vi "DAQmxTaskContainerConnect-Com-Exec.vi"(8 "error in (no error)":errorcluster, 9 "data":variant, 10 "ControlQueue":refnum<queue>, 11 "DAQmxTaksContainer_General in":refnum<class "DAQmxTaksContainer_General.lvclass">) -> (0 "error out":errorcluster, 3 "DAQmxTaksContainer_General out":refnum<class "DAQmxTaksContainer_General.lvclass">)   [LabVIEW 2018, in "DAQmxTaksContainer_General.lvclass"]
uses:
  DAQmxTaksContainer_General.lvclass
  dependecies/ControlsVIs/Clusters-def/DAQmx-Reply-Connect-client.ctl
  dependecies/ControlsVIs/Clusters-def/DAQmx-Reply-to-Connect.ctl
  dependecies/ControlsVIs/Clusters-def/SERVER-Commands.ctl
  DAQmxTask.lvclass
  Control/Control-Server/Control-Server.lvclass
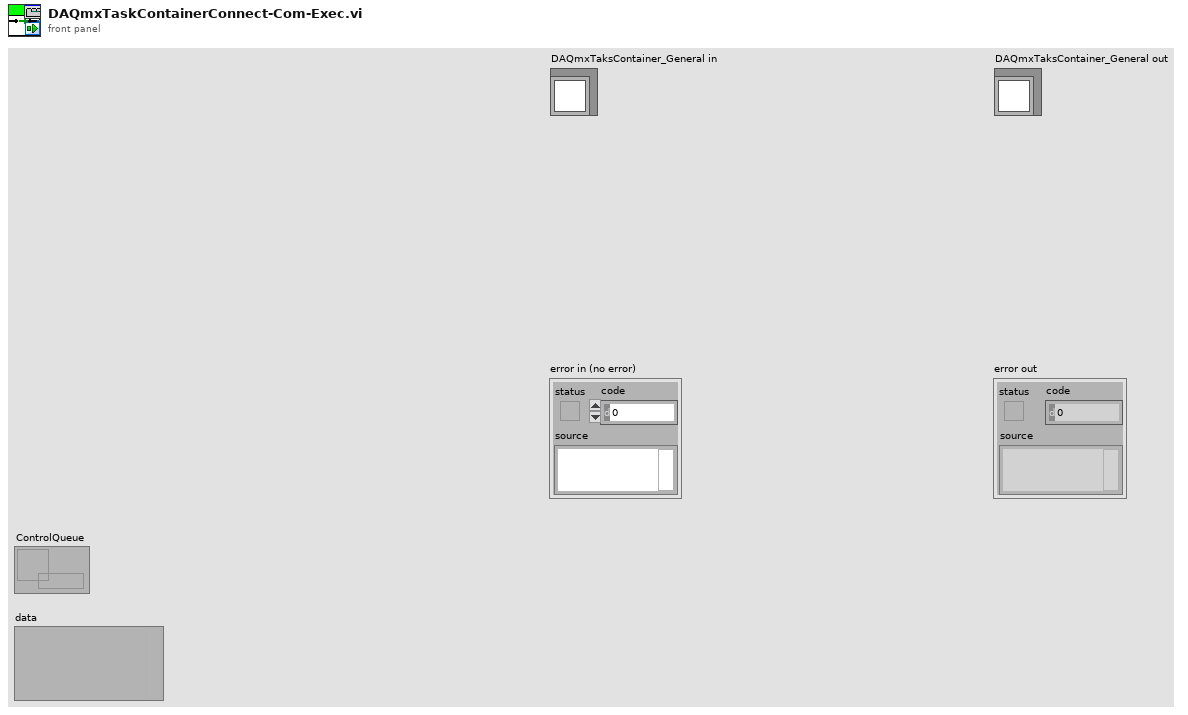
[diagram p1: front panel]
types:
  T1 = typedef "Control-Server.lvclass/SERVER-Commands.ctl" = string
  T2 = typedef "DAQmxTaksContainer_General.lvclass/DAQmx-Reply-to-Connect.ctl" = cluster{"On/Off":bool, "error":errorcluster, "DAQmxTaskContainer_General":refnum<class "DAQmxTaksContainer_General.lvclass">}
  T3 = typedef "DAQmxTaksContainer_General.lvclass/DAQmx-Reply-Connect-client.ctl" = cluster{"on/off":bool, "RelayKeyHeater/off":bool, "LaserShutter":bool, "AcceleratorShutter":bool, "Power":bool, "Faraday Cup Status":bool, "Pump Start_Stop":bool, "error":errorcluster}
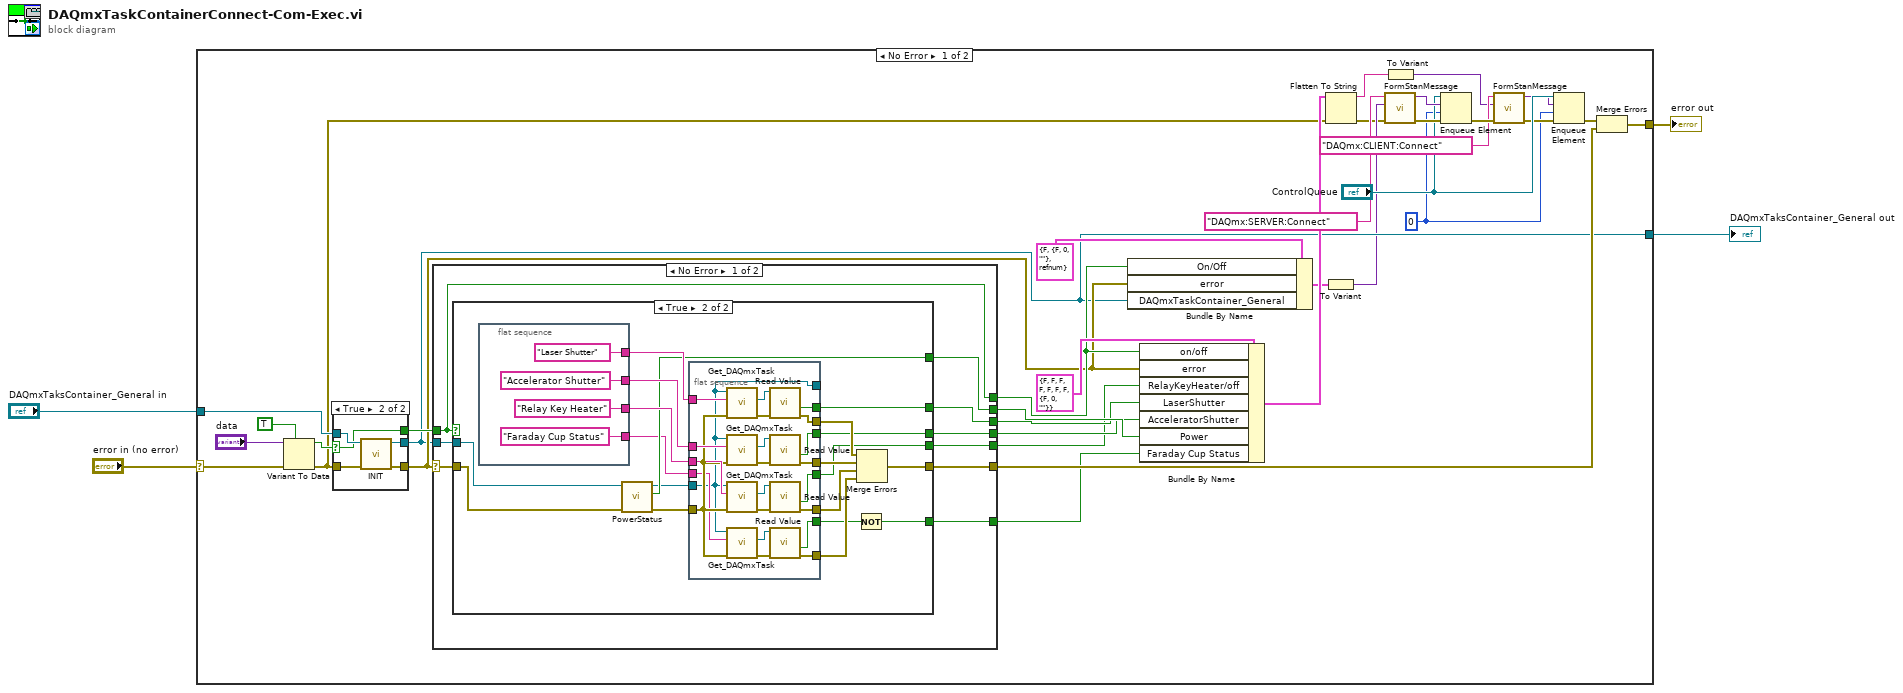
[diagram p0: block diagram]
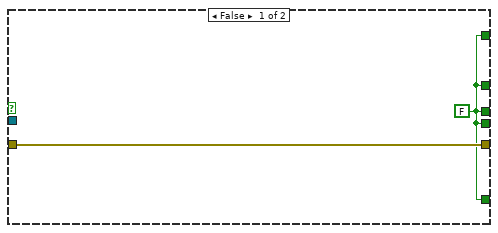
[diagram p2: hidden frame]
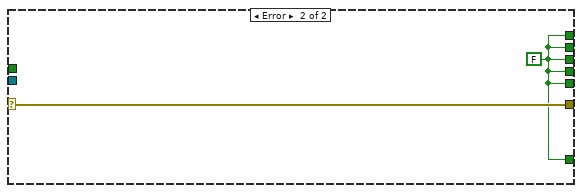
[diagram p3: hidden frame]
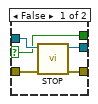
[diagram p4: hidden frame]
diagram:
  n1 = case shown="No Error" "error in (no error)" {
    selector: "error in (no error)" -> [w30 w109]
    tunnel: [w29 w109] -> w3
    tunnel: "DAQmxTaksContainer_General in" -> [w28 w108]
    tunnel: [w16 w108] -> w4
    frame No Error {
      w8 = 0 ("timeout en ms (-1)")
      n2 = Variant To Data(error in=w30, type=TRUE, Variant="data") -> (data=w37:bool, error out=w27:errorcluster)
      n3 = case shown="True" w37 {
        selector: w37 -> [w99 w104]
        tunnel: w28 -> [w102 w107]
        tunnel: [w101 w106] -> w16
        tunnel: [w100 w105] -> w17
        tunnel: [w99 w104] -> w36
        tunnel: w27 -> [w98 w103]
        frame False {
          n4 = call-dynamic "STOP.vi"("error in (no error)"=w98, "Stop in"=w102) -> ("error out"=w100:errorcluster, "Stop out"=w101:refnum<class "DAQmxTaksContainer_General.lvclass">)  [unwired: 8 in]
        }
        frame True {
          n5 = call-dynamic "INIT.vi"("error in (no error)"=w103, "DAQmxTaksContainer_General in"=w107) -> ("error out"=w105:errorcluster, "DAQmxTaksContainer_General out"=w106:refnum<class "DAQmxTaksContainer_General.lvclass">)  [unwired: 8 in]
        }
      }
      n6 = case shown="No Error" w17 {
        selector: w17 -> [w47 w97]
        tunnel: [w40 w96] -> w31
        tunnel: w36 -> [w40 _]
        tunnel: w16 -> [w48 _]
        tunnel: [w46 w97] -> w26
        tunnel: [w45 w96] -> w25
        tunnel: [w44 w96] -> w24
        tunnel: [w43 w96] -> w23
        tunnel: [w42 w96] -> w22
        tunnel: [w41 w96] -> w21
        frame No Error {
          n7 = case shown="True" w40 {
            tunnel: w48 -> [_ w57]
            tunnel: w47 -> [w50 w56]
            tunnel: [w50 w63] -> w46
            tunnel: [w49 w59] -> w45
            tunnel: [w49 w62] -> w44
            tunnel: [w49 w61] -> w43
            tunnel: [w49 w60] -> w42
            tunnel: [w49 w54] -> w41
            frame False {
              w49 = FALSE ("Data")
            }
            frame True {
              n8 = flat-sequence {
                tunnel: ["Relay Key Heater" ("Task name")] -> w66
                tunnel: ["Accelerator Shutter" ("Task name")] -> w65
                tunnel: ["Laser Shutter" ("Task name")] -> w64
                tunnel: ["Faraday Cup Status" ("Task name")] -> w55
                frame #0 {
                }
              }
              n9 = call "PowerStatus.vi"("error in (no error)"=w56, "DAQmxTaskContainer_General in"=w57) -> ("error out"=w51:errorcluster, "On/Off"=w59:bool, "DAQmxTaskContainer_General out"=w52:refnum<class "DAQmxTaksContainer_General.lvclass">)  [unwired: 7 in]
              n10 = flat-sequence {
                tunnel: [w95] -> w69
                tunnel: [w94] -> w68
                tunnel: [w93] -> w67
                tunnel: w66 -> [w92]
                tunnel: w65 -> [w91]
                tunnel: w64 -> [w90]
                tunnel: [w89] -> w62
                tunnel: [w88] -> w61
                tunnel: [w87] -> w60
                tunnel: [w86] -> w58
                tunnel: [w74] -> _
                tunnel: w51 -> [w85]
                tunnel: w55 -> [w84]
                tunnel: [w77] -> w53
                tunnel: w52 -> [w74]
                frame #0 {
                  n11 = call "Get_DAQmxTask.vi"("error in (no error)"=w85, "Task name"=w90, "DAQmxTaksContainer_General in"=w74) -> ("error out"=w78:errorcluster, "DAQmx Task"=w79:refnum<class "DAQmxTask.lvclass">)  [unwired: 6 in, 1 out]
                  n12 = call "Get_DAQmxTask.vi"("error in (no error)"=w85, "Task name"=w91, "DAQmxTaksContainer_General in"=w74) -> ("error out"=w80:errorcluster, "DAQmx Task"=w81:refnum<class "DAQmxTask.lvclass">)  [unwired: 6 in, 1 out]
                  n13 = call "Get_DAQmxTask.vi"("error in (no error)"=w85, "Task name"=w92, "DAQmxTaksContainer_General in"=w74) -> ("error out"=w82:errorcluster, "DAQmx Task"=w83:refnum<class "DAQmxTask.lvclass">)  [unwired: 6 in, 1 out]
                  n14 = call "Get_DAQmxTask.vi"("error in (no error)"=w85, "Task name"=w84, "DAQmxTaksContainer_General in"=w74) -> ("error out"=w76:errorcluster, "DAQmx Task"=w75:refnum<class "DAQmxTask.lvclass">)  [unwired: 6 in, 1 out]
                  n15 = call-dynamic "Read Value.vi"("error in (no error)"=w78, "DAQmxTask en entrée"=w79) -> ("error out"=w93:errorcluster, "Data"=w89:bool)  [unwired: 6 in, 2 out]
                  n16 = call-dynamic "Read Value.vi"("error in (no error)"=w80, "DAQmxTask en entrée"=w81) -> ("error out"=w94:errorcluster, "Data"=w88:bool)  [unwired: 6 in, 2 out]
                  n17 = call-dynamic "Read Value.vi"("error in (no error)"=w82, "DAQmxTask en entrée"=w83) -> ("error out"=w95:errorcluster, "Data"=w87:bool)  [unwired: 6 in, 2 out]
                  n18 = call-dynamic "Read Value.vi"("error in (no error)"=w76, "DAQmxTask en entrée"=w75) -> ("error out"=w86:errorcluster, "Data"=w77:bool)  [unwired: 6 in, 2 out]
                }
              }
              n19 = Not(x=w53) -> (.not. x?=w54:bool)
              n20 = Merge Errors(w67, w68, w69, w58) -> (w63:errorcluster)
            }
          }
        }
        frame Error {
          w96 = FALSE
        }
      }
      n21 = Bundle By Name(cluster=T2 {"On/Off"=FALSE, "error"={"status"=FALSE, "code"=0, "source"=""}, "DAQmxTaskContainer_General"=refnum} ("Cluster"), "On/Off"=w31, "error"=w17, "DAQmxTaskContainer_General"=w16) -> (w6:T2)
      n22 = Bundle By Name(cluster=T3 {"on/off"=FALSE, "RelayKeyHeater/off"=FALSE, "LaserShutter"=FALSE, "AcceleratorShutter"=FALSE, "Power"=FALSE, "Faraday Cup Status"=FALSE, "Pump Start_Stop"=FALSE, "error"={"status"=FALSE, "code"=0, "source"=""}} ("output cluster"), "on/off"=w31, "error"=w17, "RelayKeyHeater/off"=w22, "LaserShutter"=w24, "AcceleratorShutter"=w23, "Power"=w25, "Faraday Cup Status"=w21) -> (w34:T3)
      n23 = Flatten To String(anything=w34, error in (no error)=w27) -> (data string=w33:string, error out=w5:errorcluster)  [unwired: 2 in, 1 out]
      n24 = To Variant(anything=w6) -> (Variant=w14:variant)
      n25 = call "FormStanMessage.vi"("error in"=w5, "data"=w14, "Command"=T1 "DAQmx:SERVER:Connect" ("Commands")) -> ("error out"=w20:errorcluster, "message"=w19:variant)  [unwired: 7 in]
      n26 = To Variant(anything=w33) -> (Variant=w7:variant)
      n27 = Enqueue Element(queue="ControlQueue", element=w19, timeout in ms (-1)=w8, error in (no error)=w20) -> (error out=w11:errorcluster)  [unwired: 2 out]
      n28 = call "FormStanMessage.vi"("error in"=w11, "data"=w7, "Command"=T1 "DAQmx:CLIENT:Connect" ("Commands")) -> ("error out"=w12:errorcluster, "message"=w13:variant)  [unwired: 7 in]
      n29 = Enqueue Element(queue="ControlQueue", element=w13, timeout in ms (-1)=w8, error in (no error)=w12) -> (error out=w10:errorcluster)  [unwired: 2 out]
      n30 = Merge Errors(w10, w26) -> (w29:errorcluster)
    }
    frame Error {
    }
  }
  "error out" <- w3
  "DAQmxTaksContainer_General out" <- w4
